vi "Make DLL Param(Time).vi"(1 "Time":T2) -> (0 "pTime":T1)   [LabVIEW 8.6, in "Keyence LJ-V7000.lvlib"]
uses:
  Keyence LJ-V7000.lvlib
  Public/Clusters/Time.ctl
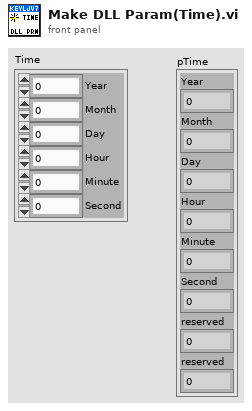
[diagram p1: front panel]
types:
  T1 = cluster{"Year":u8, "Month":u8, "Day":u8, "Hour":u8, "Minute":u8, "Second":u8, "reserved":u8, "reserved":u8}
  T2 = typedef "Keyence LJ-V7000.lvlib/Time.ctl" = cluster{"Year":u8, "Month":u8, "Day":u8, "Hour":u8, "Minute":u8, "Second":u8}
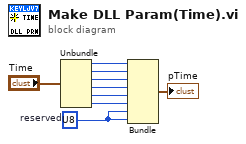
[diagram p0: block diagram]
diagram:
  w2 = u8 ?  # reserved
  n1 = Unbundle("Time") -> ("Year"=w8:u8, "Month"=w7:u8, "Day"=w6:u8, "Hour"=w5:u8, "Minute"=w4:u8, "Second"=w3:u8)
  n2 = Bundle("Year"=w8, "Month"=w7, "Day"=w6, "Hour"=w5, "Minute"=w4, "Second"=w3, "reserved"=w2, "reserved"=w2) -> (→"pTime":T1)  [unwired: 1 in]
